vi "CleanUpNode.vi"(8 "error in (no error)":errorcluster, 10 "Parameters":variant, 11 "device in":refnum<class "device.lvclass">) -> (0 "error out":errorcluster, 3 "device out":refnum<class "device.lvclass">)   [LabVIEW 2013, in "device.lvclass"]
doc: "This VI will clean any reference handled internally in the node"
uses:
  device.lvclass
  device registry command.ctl
  <vilib>/NI/Configuration Framework/Node/NISE_CEF_Node.lvclass
  device.lvclass/device.ctl
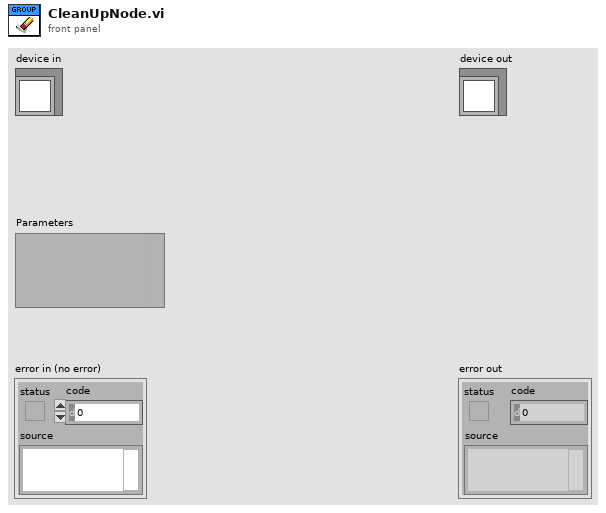
[diagram p1: front panel]
types:
  T1 = typedef "device.lvclass/device registry command.ctl" = enum16{"add device", "remove device", "get next available"}
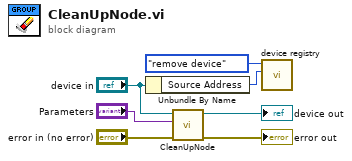
[diagram p0: block diagram]
diagram:
  n1 = Unbundle By Name("device in") -> ("Source Address"=w2:u8)
  n2 = call-parent "CleanUpNode.vi"("error in (no error)"="error in (no error)", "Parameters"="Parameters", "NISE_CEF_Node in"="device in") -> ("error out"=→"error out":errorcluster, "NISE_CEF_Node out"=→"device out":refnum<class "device.lvclass">)  [unwired: 7 in]
  n3 = call "device registry.vi"("device"=w2, "command"=device_registry_command."remove device") -> ()  [unwired: 8 in, 2 out]
